vi "Get Status.vi"(8 "error in (no error)":errorcluster, 11 "Statnett C37.118 DLL in":refnum<class "Statnett C37.118 DLL.lvclass">) -> (0 "error out":errorcluster, 1 "Configuration File Received":bool, 2 "Timeout":bool, 3 "Statnett C37.118 DLL out":refnum<class "Statnett C37.118 DLL.lvclass">, 4 "Configuration Read OK":bool, 5 "PDC Connected":bool)   [LabVIEW 2013, in "PMU Recorder Light.lvlib" / "Statnett C37.118 DLL.lvclass"]
uses:
  Statnett C37.118 DLL.lvclass
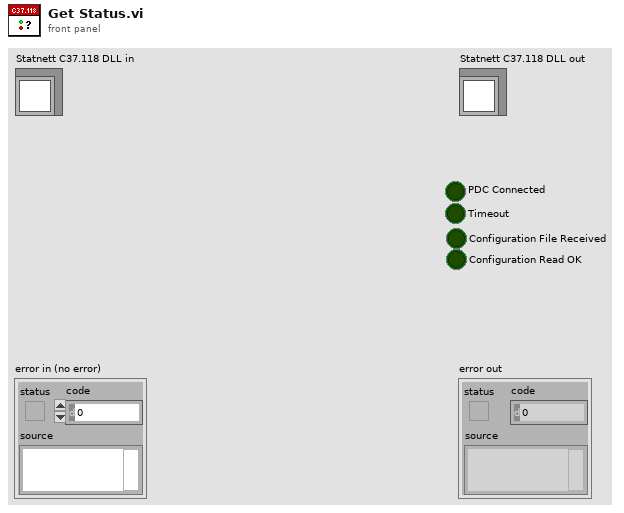
[diagram p1: front panel]
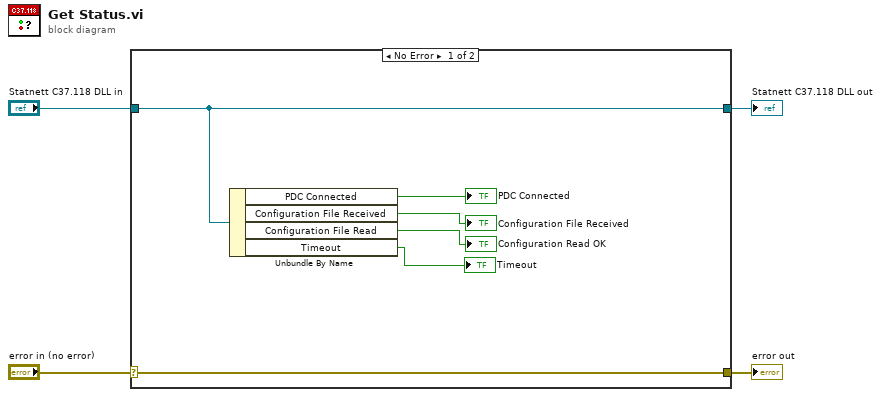
[diagram p0: block diagram]
diagram:
  n1 = case shown="No Error" "error in (no error)" {
    selector: "error in (no error)" -> [w10 w12]
    tunnel: [w10 w12] -> w3
    tunnel: [w9 w11] -> w1
    tunnel: "Statnett C37.118 DLL in" -> [w9 w11]
    frame No Error {
      n2 = Unbundle By Name(w9) -> ("PDC Connected"=→"PDC Connected":bool, "Configuration File Received"=→"Configuration File Received":bool, "Configuration File Read"=→"Configuration Read OK":bool, "Timeout"=→"Timeout":bool)
    }
    frame Error {
    }
  }
  "error out" <- w3
  "Statnett C37.118 DLL out" <- w1
